vi "create test channels.vi"() -> (0 "error out":errorcluster, 1 "names":string[](array[string]), 2 "chans":refnum<class "TBM channel.lvclass">[](array[class]), 3 "TDMS datalogger configuration out":refnum<class "Binary datalogger configuration.lvclass">)   [LabVIEW 2013, in "Binary logger tests.lvlib"]
uses:
  Binary logger tests.lvlib
  <vilib>/NI/Tag Bus Module Framework/channel/TBM channel.lvclass
  configuration/Binary datalogger configuration.lvclass
  <vilib>/NI/Tag Bus Module Framework/channel/channel classification.ctl
  <vilib>/NI/Tag Bus/tag/tag descriptor.lvclass/tag descriptor.ctl
  configuration/Binary datalogger configuration.lvclass/Binary datalogger configuration.ctl
  <vilib>/NI/Tag Bus/tag/write raw default value.vi
  configuration/Write queue size.vi
  configuration/Write scans per write.vi
  configuration/Write backup directory.vi
  configuration/Write Path.vi
  <vilib>/NI/Configuration Framework/serializable configuration/NISE_CEF_serializable configuration.lvclass
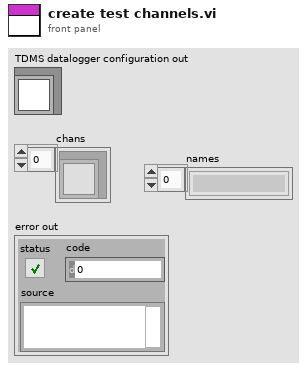
[diagram p1: front panel]
types:
  T1 = typedef "tag bus.lvlib/tag descriptor.lvclass/Data Type.ctl" = enum16{"Double", "Single", "I64", "I32", "I16", "I8", "U64", "U32", "U16", "U8", "Boolean", "String", "Array of Double", "Array of Single", "Array of I64", "Array of I32", "Array of I16", "Array of I8", "Array of U64", "Array of U32", "Array of U16", "Array of U8", "Array of Boolean", "Array of String"}
  T2 = typedef "TBM channel.lvclass/channel classification.ctl" = enum16{"input data", "output data", "processing parameter", "processing result"}
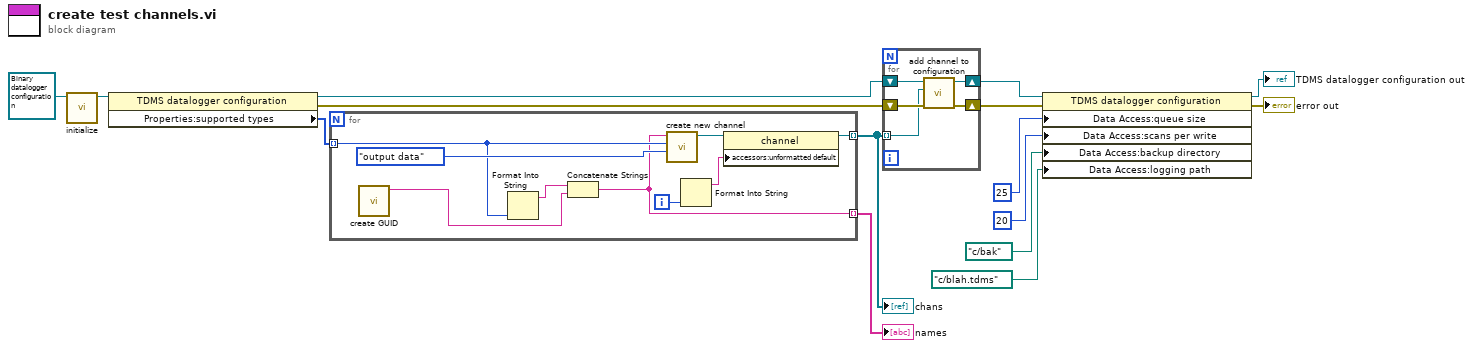
[diagram p0: block diagram]
diagram:
  n1 = call <vilib>:"initialize.vi"("configuration in"=refnum<class "Binary datalogger configuration.lvclass"> refnum ("TDMS datalogger configuration")) -> ("configuration out"=w10:refnum<class "Binary datalogger configuration.lvclass">)  [unwired: 8 in, 2 out]
  n2 = property class="TDMS datalogger configuration"(reference=w10) -> (reference out=w13:refnum<class "Binary datalogger configuration.lvclass">, error out=w14:errorcluster, "Properties:supported types"=w11:T1[])  [unwired: 1 in]
  n3 = for {
    tunnel: [w22] -> w15 mode=indexing
    tunnel: w11 -> [w19] mode=indexing
    tunnel: [w16] -> w9 mode=indexing
    i -> [w21]
    n4 = call <vilib>:"create GUID.vi"() -> ("uuid"=w18:string)  [unwired: 10 in, 1 out]
    n5 = Format Into String(w19) -> (resulting string=w17:string)  [unwired: 3 in, 1 out]
    n6 = Concatenate Strings(w17, w18) -> (w16:string)
    n7 = call <vilib>:"create new channel.vi"("channel classification"=channel_classification."output data", "data type"=w19, "channel name"=w16) -> ("channel"=w24:refnum<class "TBM channel.lvclass">)  [unwired: 8 in]
    n8 = Format Into String(w21) -> (resulting string=w20:string)  [unwired: 3 in, 1 out]
    n9 = property class="channel"(reference=w24, "accessors:unformatted default"=w20) -> (reference out=w22:refnum<class "TBM channel.lvclass">)  [unwired: 1 in, 1 out]
  }
  "chans" <- w15
  "names" <- w9
  n10 = for {
    shift-right: [w28] -> w4
    shift-left: w13 -> [w29]
    shift-right: [w26] -> w1
    shift-left: w14 -> [w27]
    tunnel: w15 -> [w25] mode=indexing
    n11 = call "add channel to configuration.vi"("error in"=w27, "TBM channel in"=w25, "bin datalogger configuration in"=w29) -> ("error out"=w26:errorcluster, "bin datalogger configuration out"=w28:refnum<class "Binary datalogger configuration.lvclass">)  [unwired: 7 in]
  }
  n12 = property class="TDMS datalogger configuration"(reference=w4, error in=w1, "Data Access:queue size"=25 ("queue size"), "Data Access:scans per write"=20 ("scans per write"), "Data Access:backup directory"=path "c:/bak" ("backup directory"), "Data Access:logging path"=path "c:/blah.tdms" ("logging path")) -> (reference out=→"TDMS datalogger configuration out":refnum<class "Binary datalogger configuration.lvclass">, error out=→"error out":errorcluster)
